vi "Create.vi"(8 "error in (no error)":errorcluster, 10 "Waveform Settings":T1, 11 "Waveform Factory in":refnum<class "Waveform Factory.lvclass">) -> (0 "error out":errorcluster, 2 "Waveform":refnum<class "Waveform.lvclass">, 3 "Waveform Factory out":refnum<class "Waveform Factory.lvclass">)   [LabVIEW 2015, in "Waveform Factory.lvclass"]
uses:
  Waveform Factory.lvclass
  Waveform Generator/Waveform Generator.lvclass
  Waveform/Waveform.lvclass
  Typedefs/Waveform Types.ctl
  Typedefs/FAMT Typedefs.lvlib
  Typedefs/Waveform Settings.ctl
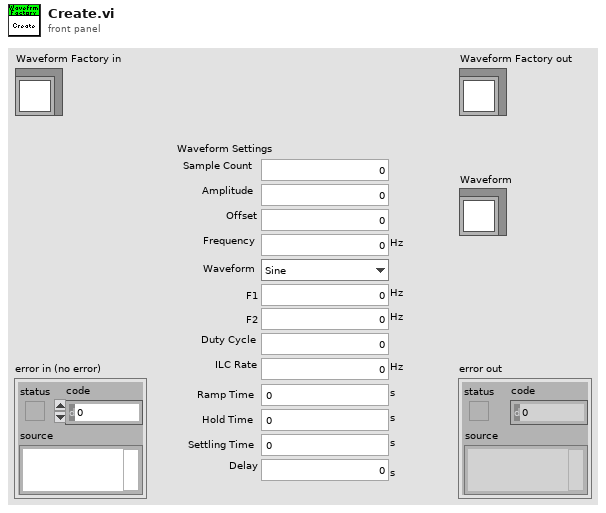
[diagram p1: front panel]
types:
  T1 = typedef "FAMT Typedefs.lvlib/Waveform Settings.ctl" = cluster{"Sample Count":u32, "Amplitude":dbl, "Offset":dbl, "Frequency":dbl[unit], "Waveform":T2, "F1":dbl[unit], "F2":dbl[unit], "Duty Cycle":dbl, "ILC Rate":dbl[unit], "Ramp Time":dbl[unit], "Hold Time":dbl[unit], "Settling Time":dbl[unit], "Delay":dbl[unit]}
  T2 = typedef "FAMT Typedefs.lvlib/Waveform Types.ctl" = enum16{"Sine", "Triangle", "Square", "Sawtooth", "Chirp", "Gaussian", "Trapezoid"}
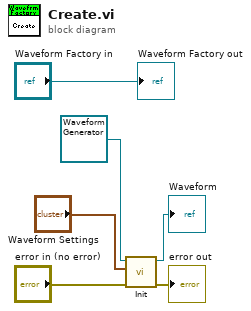
[diagram p0: block diagram]
diagram:
  n1 = call "Init.vi"("error in (no error)"="error in (no error)", "Waveform Settings"="Waveform Settings", "Waveform Generator in"=refnum<class "Waveform Generator.lvclass"> refnum ("Waveform Generator.lvclass")) -> ("error out"=→"error out":errorcluster, "Waveform Generator out"=→"Waveform":refnum<class "Waveform Generator.lvclass">)  [unwired: 7 in]
  "Waveform Factory out" <- "Waveform Factory in"
